vi "Rotation.vi"() -> ()   [LabVIEW 2018]
doc: "Rotation: This example is a rotation example that can perform basic geometric transformations on collected images, referring to rotating objects or images at a certain angle around a central point."
uses:
  vi.lib/VIRobotics/opencv_yiku/ctls/Point2f.ctl
  vi.lib/VIRobotics/opencv_yiku/ctls/Size.ctl
  vi.lib/VIRobotics/opencv_yiku/Mat/Mat_32F/Mat_32F.lvclass
  D:/Program Files/company/National Instruments/LabVIEW 2018/vi.lib/addons/VIRobotics/opencv_yiku/Mat/Mat/Mat.lvclass
  vi.lib/VIRobotics/opencv_yiku/Mat/Mat_8U/Mat_8U.lvclass
  vi.lib/VIRobotics/opencv_yiku/Mat/Create_Mat_32F.vi
  vi.lib/VIRobotics/opencv_yiku/Cap/Cap.lvclass
  vi.lib/VIRobotics/opencv_yiku/opencv_yiku.lvlib
panel:
  out "new picture 2":picture
  in  "stop":bool
  out "new picture":picture
  # "Overview: Demonstrates how to rotates the image by some degree with respect to center without any scaling.\nRequirements: Windows.\nInstructions: \n1.Make sure your computer has a camera.\n2.Run the VI."
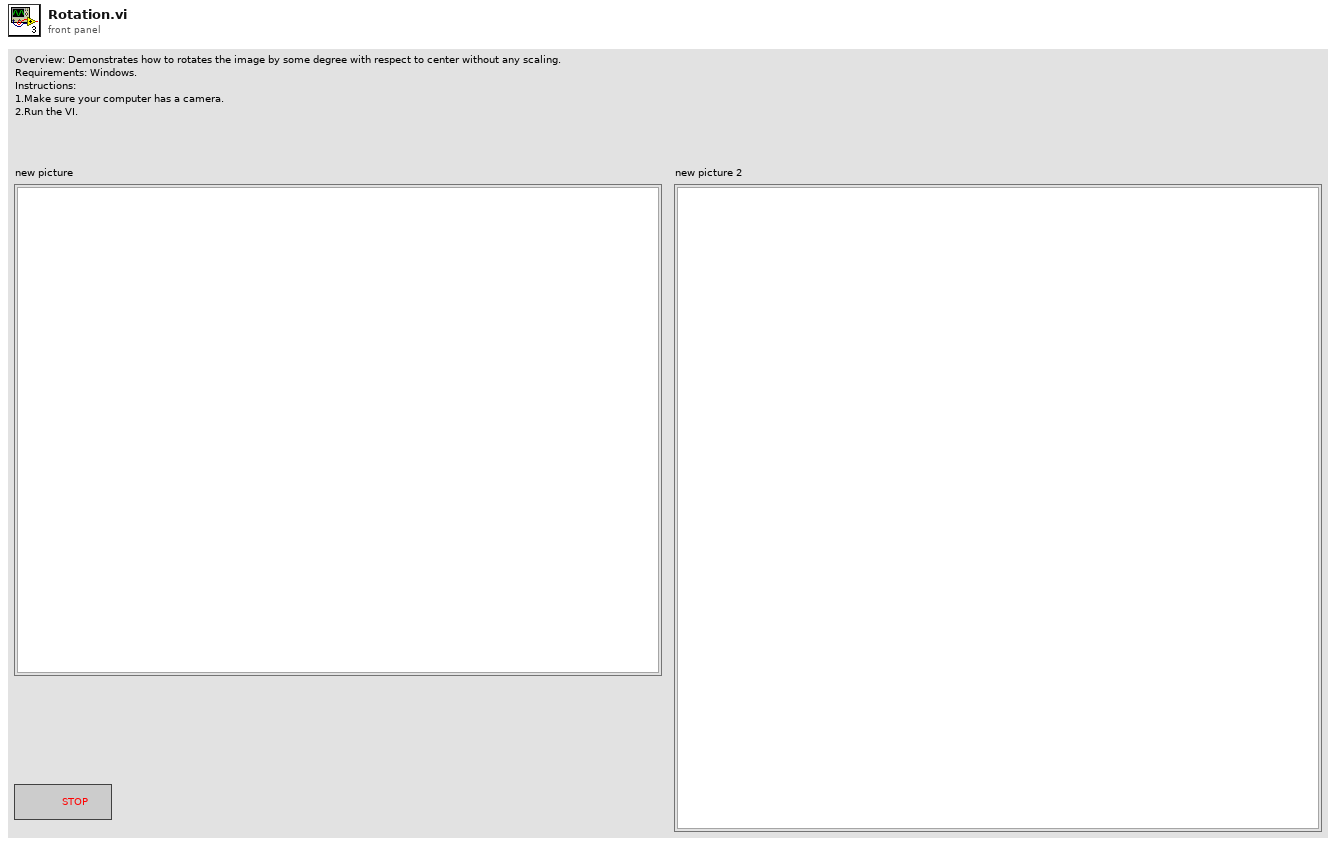
[diagram p1: front panel]
types:
  T1 = typedef "opencv_yiku.lvlib/Point2f.ctl" = cluster{"x":sgl, "y":sgl}
  T2 = typedef "opencv_yiku.lvlib/Size.ctl" = cluster{"x":i32, "y":i32}
  T3 = enum16{"COLOR_BGR2BGRA", "COLOR_BGRA2BGR", "COLOR_BGR2RGBA", "COLOR_RGBA2BGR", "COLOR_BGR2RGB", "COLOR_BGRA2RGBA", "COLOR_BGR2GRAY", "COLOR_RGB2GRAY", "COLOR_GRAY2BGR", "COLOR_GRAY2BGRA"}
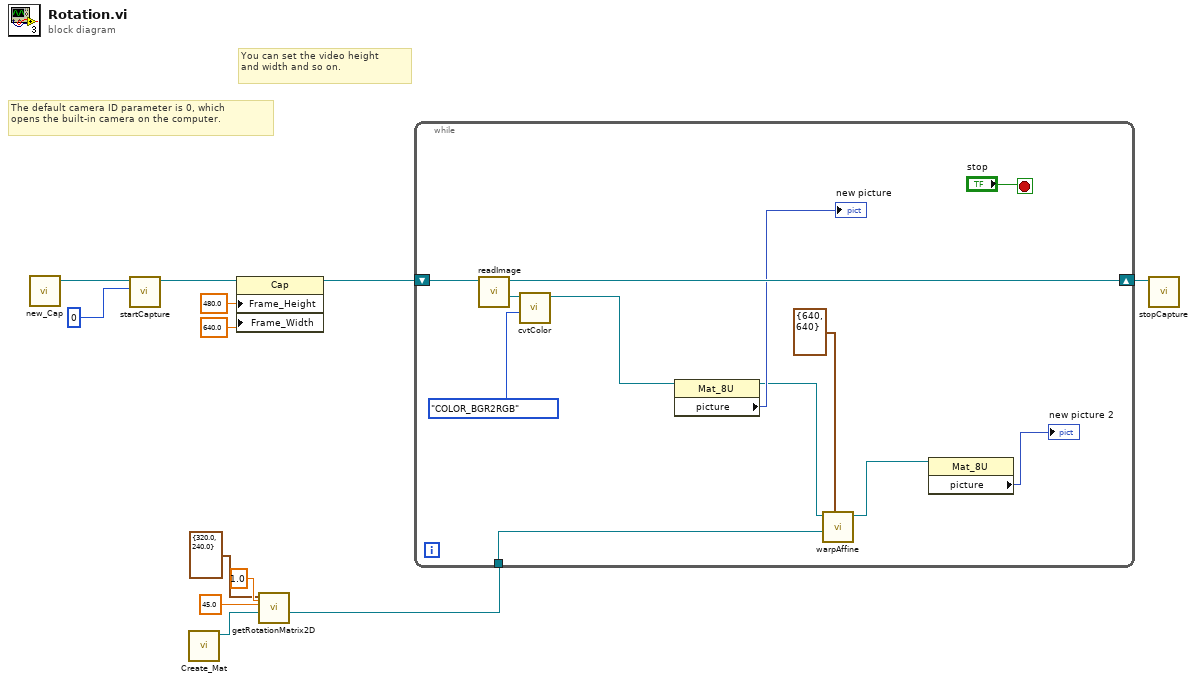
[diagram p0: block diagram]
diagram:
  # "The default camera ID parameter is 0, which \nopens the built-in camera on the computer."
  # "You can set the video height \nand width and so on."
  n1 = call "new_Cap.vi"() -> ("Cap out"=w12:refnum<class "Cap.lvclass">)  [unwired: 10 in, 1 out]
  n2 = call "startCapture.vi"("cameraID"=0, "Cap in"=w12) -> ("Cap out"=w9:refnum<class "Cap.lvclass">)  [unwired: 8 in, 1 out]
  n3 = call-poly "Create_Mat.vi"() -> ("Mat_32F_out"=w5:refnum<class "Mat_32F.lvclass">)  [unwired: 10 in, 1 out]
  n4 = property class="Cap"(reference=w9, "Frame_Height"=480.0, "Frame_Width"=640.0) -> (reference out=w8:refnum<class "Cap.lvclass">)  [unwired: 1 in, 1 out]
  n5 = call "getRotationMatrix2D.vi"("scale"=1.0, "dst in"=w5, "angle"=45.0, "Centre"=T1 {"x"=320.0, "y"=240.0}) -> ("dst out"=w1:refnum<class "Mat_32F.lvclass">)  [unwired: 6 in, 1 out]
  n6 = while {
    shift-right: [w23] -> w10
    shift-left: w8 -> [w24]
    tunnel: w1 -> [w16]
    stop <- "stop" stop-if-true
    n7 = call "readImage.vi"("Cap in"=w24) -> ("Mat out"=w21:refnum<class "Mat_8U.lvclass">, "Cap out"=w23:refnum<class "Cap.lvclass">)  [unwired: 8 in, 1 out]
    n8 = call "cvtColor.vi"("dstCn"=T3."COLOR_BGR2RGB", "src"=w21) -> ("src out"=w18:refnum<class "Mat_8U.lvclass">)  [unwired: 7 in, 2 out]
    n9 = property class="Mat_8U"(reference=w18) -> (reference out=w17:refnum<class "Mat_8U.lvclass">, "picture"=→"new picture":picture)  [unwired: 1 in, 1 out]
    n10 = call "warpAffine.vi"("Size"=T2 {"x"=640, "y"=640}, "M"=w16, "Mat in"=w17) -> ("dst out"=w14:refnum<class "Mat_8U.lvclass">)  [unwired: 7 in, 1 out]
    n11 = property class="Mat_8U"(reference=w14) -> ("picture"=→"new picture 2":picture)  [unwired: 1 in, 2 out]
  }
  n12 = call "stopCapture.vi"("Cap in"=w10) -> ()  [unwired: 10 in, 1 out]
